vi "Parse Boolean.vi"(11 "stream in":u8[](array[numeric])) -> (0 "Value":bool, 3 "stream out":u8[](array[numeric]))   [LabVIEW 2015]
doc: "Read (one byte) boolean value from a UART data stream."
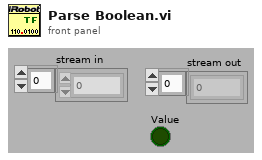
[diagram p1: front panel]
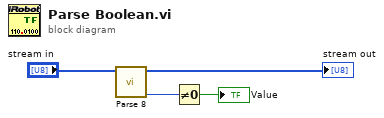
[diagram p0: block diagram]
diagram:
  n1 = call "Parse 8.vi"("stream in"="stream in") -> ("value"=w1:u8, "stream out"=→"stream out":u8[])  [unwired: 9 out]
  n2 = Not Equal To 0?(x=w1) -> (x != 0?=→"Value":bool)
